vi "Math Test Suite.vi"() -> ()   [LabVIEW 2009]
doc: "This example demonstrates how to programmatically save the test report to a file."
uses:
  classes/Test Suite/Test Suite.lvclass
panel:
  in  "error in (no error)":errorcluster
  out "error out":errorcluster
  # "See block diagram"
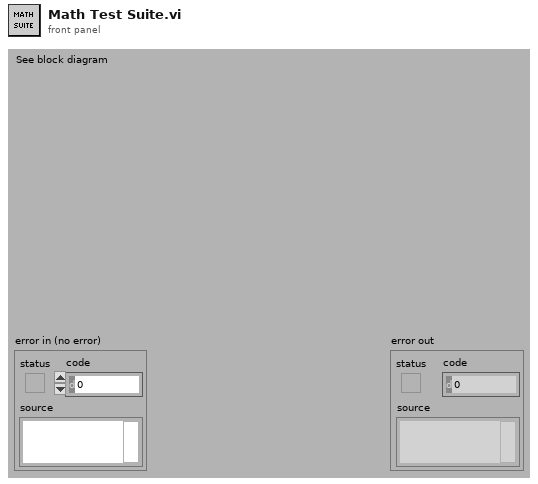
[diagram p1: front panel]
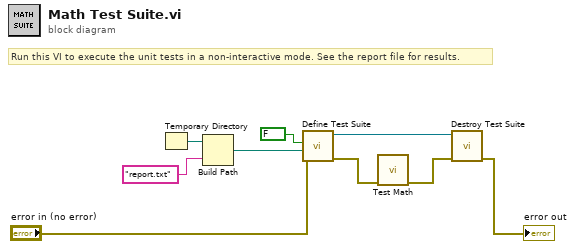
[diagram p0: block diagram]
diagram:
  # "Run this VI to execute the unit tests in a non-interactive mode. See the report file for results."
  n1 = Temporary Directory() -> (w4:path)
  n2 = Build Path(base path=w4, name or relative path="report.txt") -> (appended path=w2:path)
  n3 = call "Define Test Suite.vi"("error in (no error)"="error in (no error)", "Report Path"=w2, "Interactive"=FALSE) -> ("error out"=w9:errorcluster, "Test Suite"=w7:refnum<class "Test Suite.lvclass">)  [unwired: 7 in]
  n4 = call "Test Math.vi"("error in (no error)"=w9) -> ("error out"=w8:errorcluster)  [unwired: 10 in]
  n5 = call-dynamic "Destroy Test Suite.vi"("error in (no error)"=w8, "Test Suite in"=w7) -> ("error out"=→"error out":errorcluster)  [unwired: 9 in]
